vi "display_7s.vi"(0 "Bit Restante B":bool, 1 "MSB A":bool, 4 "LSB B":bool, 5 "MSB B":bool, 6 "Bit Restante A":bool, 7 "LSB A":bool) -> (2 "output variable 2":i32, 3 "output variable":i32)   [LabVIEW 2021]
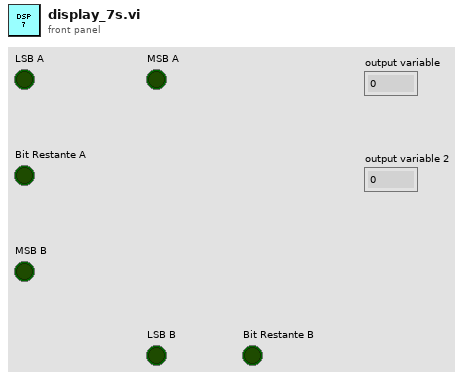
[diagram p1: front panel]
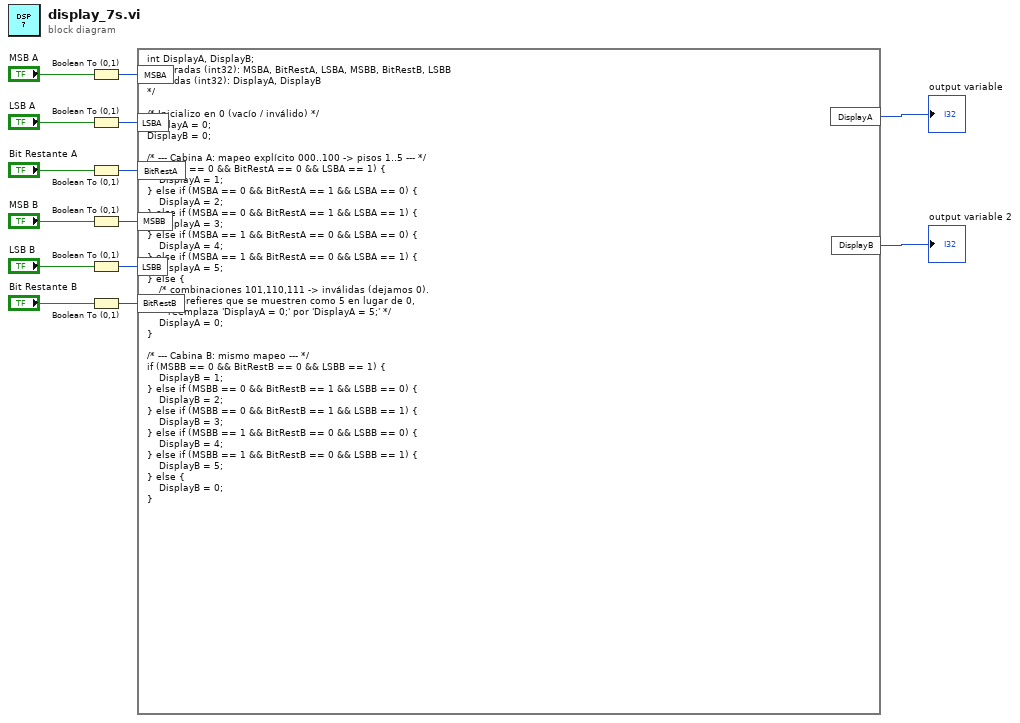
[diagram p0: block diagram]
diagram:
  n1 = Boolean To (0,1)(Boolean="MSB A") -> (0, 1=w1:i16)
  n2 = Boolean To (0,1)(Boolean="LSB A") -> (0, 1=w6:i16)
  n3 = Boolean To (0,1)(Boolean="Bit Restante A") -> (0, 1=w5:i16)
  n4 = Boolean To (0,1)(Boolean="MSB B") -> (0, 1=w4:i16)
  n5 = Boolean To (0,1)(Boolean="LSB B") -> (0, 1=w3:i16)
  n6 = Boolean To (0,1)(Boolean="Bit Restante B") -> (0, 1=w2:i16)
  n7 = formula code="int DisplayA, DisplayB;\n/* Entradas (int32): MSBA, BitRestA, LSBA, MSBB, BitRestB, LSBB\n   Salidas (int32): DisplayA, DisplayB\n*/\n\n/* Inicializo en 0 (vacío / inválido) */\nDisplayA = 0;\nDisplayB = 0;\n\n/* --- Cabina A: mapeo explícito 000..100 -> pisos 1..5 --- */\nif (MSBA == 0 && BitRestA == 0 && LSBA == 1) {\n    DisplayA = 1;\n} else if (MSBA == 0 && BitRestA == 1 && LSBA == 0) {\n    DisplayA = 2;\n} else if (MSBA == 0 && BitRestA == 1 && LSBA == 1) {\n    DisplayA = 3;\n} else if (MSBA == 1 && BitRestA == 0 && LSBA == 0) {\n    DisplayA = 4;\n} else if (MSBA == 1 && BitRestA == 0 && LSBA == 1) {\n    DisplayA = 5;\n} else {\n    /* combinaciones 101,110,111 -> inválidas (dejamos 0).\n       Si prefieres que se muestren como 5 en lugar de 0,\n       reemplaza 'DisplayA = 0;' por 'DisplayA = 5;' */\n    DisplayA = 0;\n}\n\n/* --- Cabina B: mismo mapeo --- */\nif (MSBB == 0 && BitRestB == 0 && LSBB == 1) {\n    DisplayB = 1;\n} else if (MSBB == 0 && BitRestB == 1 && LSBB == 0) {\n    DisplayB = 2;\n} else if (MSBB == 0 && BitRestB == 1 && LSBB == 1) {\n    DisplayB = 3;\n} else if (MSBB == 1 && BitRestB == 0 && LSBB == 0) {\n    DisplayB = 4;\n} else if (MSBB == 1 && BitRestB == 0 && LSBB == 1) {\n    DisplayB = 5;\n} else {\n    DisplayB = 0;\n}"("MSBA"=w1, "LSBA"=w6, "BitRestA"=w5, "MSBB"=w4, "LSBB"=w3, "BitRestB"=w2) -> ("DisplayA"=→"output variable":i32, "DisplayB"=→"output variable 2":i32)
